vi "Calibrate Gear Position.vi"(7 "CaliPosition_Bypass Calibration":bool, 9 "Offset":dbl=-3.8588, 10 "Coeff":dbl=1.1858, 11 "Gear Position":dbl) -> (3 "Calibrated Gear Position":dbl)   [LabVIEW 2018]
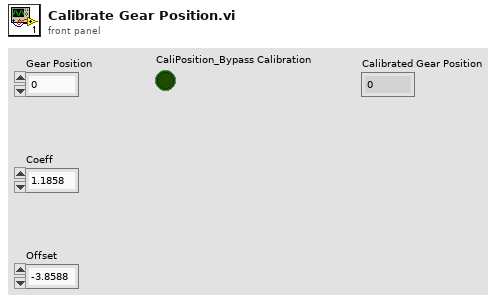
[diagram p1: front panel]
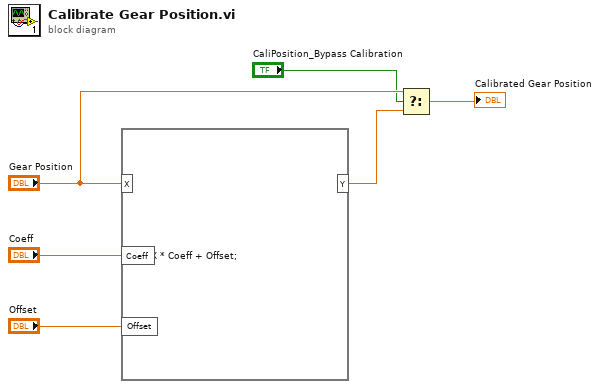
[diagram p0: block diagram]
diagram:
  n1 = formula code="Y = X * Coeff + Offset;"("X"="Gear Position", "Coeff"="Coeff", "Offset"="Offset") -> ("Y"=w4:dbl)
  n2 = Select(t="Gear Position", s="CaliPosition_Bypass Calibration", f=w4) -> (s? t:f=→"Calibrated Gear Position":dbl)
